vi "S2DS_Pop-Up Message.vi"(9 "Send mail?":bool) -> ()   [LabVIEW 2025]
uses:
  <vilib>/Utility/sysdir.llb/System Directory Type.ctl
  <vilib>/Utility/config.llb/Write Key (Boolean).vi
  <vilib>/Utility/config.llb/Write Key (String).vi
  <vilib>/Utility/config.llb/Read Key (Path).vi
  <vilib>/Utility/config.llb/NI_LVConfig.lvlib
panel:
  out "Secondary message":string
  out "Main message":string
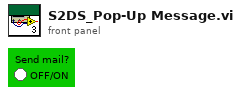
[diagram p1: front panel]
types:
  T1 = enum16{"open", "replace", "create", "open or create", "replace or create", "replace or create with confirmation"}
  T2 = typedef "System Directory Type.ctl" = i32
  T3 = typedef "NI_LVConfig.lvlib/Config Data RefNum.ctl" = refnum<k1>
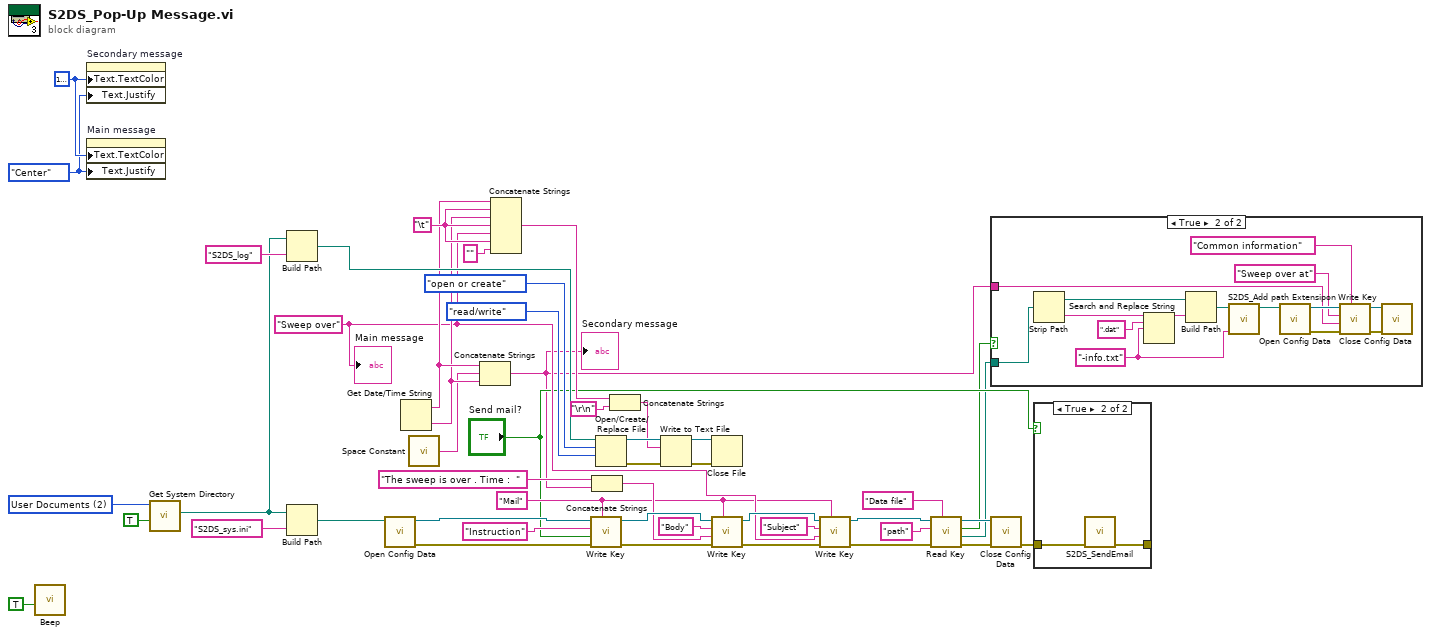
[diagram p0: block diagram]
diagram:
  w15 = "Mail" ("section")
  w48 = u32 16777224 ("Text.Text Colors:Text Color")
  w16 = "Sweep over"
  w33 = "\t"
  w46 = T2 2 items=["User Home"=0, "User Desktop"=1, "User Documents"=2, "User Application Data"=3, "User Preferences"=4, "User Temporary"=5, "Public Documents"=6, "Public Application Data"=7, "Public Preferences"=8, "Public Cache"=13, "System Core Libraries"=9, "System Installed Libraries"=10, "Application Files"=11, "Boot Volume Root"=12] ("system directory type")
  w47 = enum16{"Left", "Center", "Right"}."Center" ("Text.Justification")
  n1 = call <vilib>:"Beep.vi"("use system alert? (T)"=TRUE) -> ()  [unwired: 11 in]
  n2 = property on="Secondary message" class="Str"("Text.TextColor"=w48, "Text.Justify"=w47) -> ()  [unwired: 2 in, 2 out]
  n3 = property on="Main message" class="Str"("Text.TextColor"=w48, "Text.Justify"=w47) -> ()  [unwired: 2 in, 2 out]
  n4 = call <vilib>:"Get System Directory.vi"("create directory if not found? (F)"=TRUE, "system directory type"=w46) -> ("system directory"=w27:path)  [unwired: 9 in]
  n5 = Build Path(base path=w27, name or relative path="S2DS_log") -> (appended path=w43:path)
  n6 = Build Path(base path=w27, name or relative path="S2DS_sys.ini") -> (appended path=w25:path)
  n7 = call <vilib>:"Open Config Data.vi"("configuration file path"=w25) -> ("error out"=w12:errorcluster, "refnum"=w24:T3)  [unwired: 8 in, 1 out]
  n8 = Get Date/Time String() -> (date string=w32:string, time string=w29:string)  [unwired: 3 in]
  n9 = call <vilib>:"Space Constant.vi"() -> ("String"=w28:string)
  n10 = Concatenate Strings(w32, w28, w29) -> (w1:string)
  "Secondary message" <- w1
  n11 = Concatenate Strings(w32, w33, w29, w33, w16, w33, "" ("Error message in")) -> (w36:string)
  n12 = call-poly <vilib>:"Write Key.vi"("section"=w15, "error in (no error)"=w12, "value"="Send mail?", "key"="Instruction", "refnum"=w24) -> ("error out"=w14:errorcluster, "refnum out"=w22:T3)  [unwired: 4 in, 1 out]
  n13 = Concatenate Strings("The sweep is over . Time :  " ("string"), w1) -> (w19:string)
  n14 = Open/Create/Replace File(file path (use dialog)=w43, operation (0:open)=T1."open or create", access (0:read/write)=enum16{"read/write", "read-only", "write-only"}."read/write") -> (refnum out=w40:refnum<file>, error out=w39:errorcluster)  [unwired: 3 in, 1 out]
  n15 = Concatenate Strings(w36, "\r\n") -> (w34:string)
  n16 = Write to Text File(file (use dialog)=w40, text=w34, error in=w39) -> (refnum out=w38:refnum<file>, error out=w37:errorcluster)  [unwired: 1 in, 1 out]
  n17 = Close File(refnum=w38, error in=w37) -> ()  [unwired: 2 out]
  n18 = call-poly <vilib>:"Write Key.vi"("section"=w15, "error in (no error)"=w14, "value"=w19, "key"="Body", "refnum"=w22) -> ("error out"=w13:errorcluster, "refnum out"=w18:T3)  [unwired: 4 in, 1 out]
  n19 = call-poly <vilib>:"Write Key.vi"("section"=w15, "error in (no error)"=w13, "value"=w16, "key"="Subject", "refnum"=w18) -> ("error out"=w3:errorcluster, "refnum out"=w9:T3)  [unwired: 4 in, 1 out]
  n20 = call-poly <vilib>:"Read Key.vi"("section"="Data file", "error in (no error)"=w3, "key"="path", "refnum"=w9) -> ("error out"=w2:errorcluster, "value"=w4:path, "found?"=w5:bool, "refnum out"=w8:T3)  [unwired: 4 in]
  n21 = case shown="True" w5 {
    tunnel: w4 -> [_ w57]
    tunnel: w1 -> [_ w51]
    frame False {
    }
    frame True {
      w62 = "-info.txt" ("name or relative path")
      n22 = Strip Path(path=w57) -> (stripped path=w63:path, name=w60:string)
      n23 = Search and Replace String(input string=w60, search string=".dat", replace string=w62) -> (result string=w61:string)  [unwired: 5 in, 3 out]
      n24 = Build Path(base path=w63, name or relative path=w61) -> (appended path=w58:path)
      n25 = call "S2DS_Add path Extensipon.vi"("Extension"=w62, "path"=w58) -> ("Path"=w56:path)  [unwired: 9 in]
      n26 = call <vilib>:"Open Config Data.vi"("configuration file path"=w56) -> ("error out"=w54:errorcluster, "refnum"=w55:T3)  [unwired: 8 in, 1 out]
      n27 = call-poly <vilib>:"Write Key.vi"("section"="Common information", "error in (no error)"=w54, "value"=w51, "key"="Sweep over at", "refnum"=w55) -> ("error out"=w49:errorcluster, "refnum out"=w50:T3)  [unwired: 4 in, 1 out]
      n28 = call <vilib>:"Close Config Data.vi"("error in (no error)"=w49, "refnum"=w50) -> ()  [unwired: 8 in, 2 out]
    }
  }
  n29 = call <vilib>:"Close Config Data.vi"("error in (no error)"=w2, "refnum"=w8) -> ("error out"=w11:errorcluster)  [unwired: 8 in, 1 out]
  n30 = case shown="True" "Send mail?" {
    tunnel: w11 -> [w64 w66]
    tunnel: [w64 w65] -> _
    frame False {
    }
    frame True {
      n31 = call "S2DS_SendEmail.vi"("error in (no error)"=w66) -> ("error out"=w65:errorcluster)  [unwired: 10 in]
    }
  }
  "Main message" <- w16
